vi "Status-Query SESR.vi"(8 "error in (no error)":errorcluster, 11 "VISA resource name":refnum<visa-resource-name>) -> (0 "error out":errorcluster, 1 "standard event status register":bool[](array[boolean]), 3 "VISA resource name out":refnum<visa-resource-name>)   [LabVIEW 2016, in "Agilent 415X Series.lvlib"]
doc: "This VI returns the bits in the instrument's IEEE-488.2 Standard Event Status Register. Reading the register clears it."
uses:
  Agilent 415X Series.lvlib
panel:
  # "OPC  RQC  QYE  DDE   EXE  CME     -      PON"
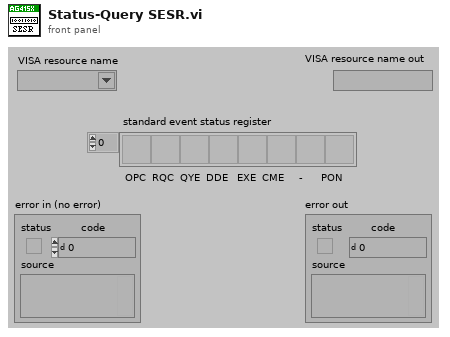
[diagram p1: front panel]
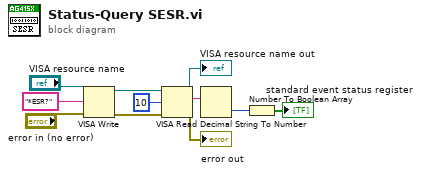
[diagram p0: block diagram]
diagram:
  n1 = VISA Write(VISA resource name="VISA resource name", write buffer="*ESR?", error in (no error)="error in (no error)") -> (VISA resource name out=w5:refnum<visa-resource-name>, error out=w6:errorcluster)  [unwired: 1 out]
  n2 = VISA Read(VISA resource name=w5, byte count=u32 10, error in (no error)=w6) -> (VISA resource name out=→"VISA resource name out":refnum<visa-resource-name>, read buffer=w9:string, error out=→"error out":errorcluster)  [unwired: 1 out]
  n3 = Decimal String To Number(string=w9) -> (number=w1:i32)  [unwired: 2 in, 1 out]
  n4 = Number To Boolean Array(number=w1) -> (Boolean array=→"standard event status register":bool[])
